vi "Controlling_the_Pump_Reglo_D.vi"(5 "Parameter":string, 7 "Command":T1=enum."Start Reglo Digital", 8 "error in (no error)":errorcluster, 11 "Pumpe":T2=enum."P_01") -> (0 "error out":errorcluster, 3 "Answer":string)   [LabVIEW 2019]
doc: "Contains the commands to controll the Reglo Digital\n\n08.12.2003 - Ismatec/CS"
uses:
  Pumpen.ctl
  Controlling_the_Pump_Reglo_D.ctl
panel:
  in  "VISA resource name In":refnum<visa-resource-name>="COM1"
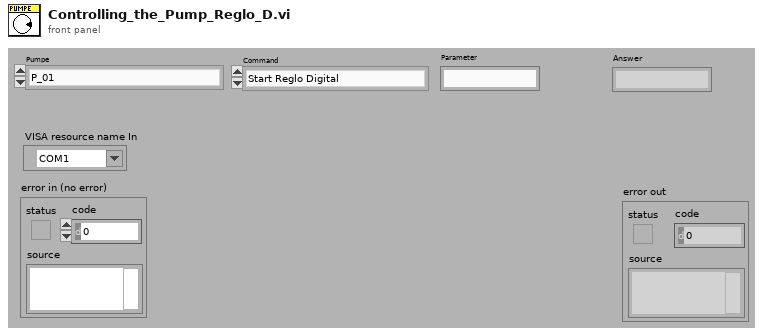
[diagram p1: front panel]
types:
  T1 = typedef "Controlling_the_Pump_Reglo_D.ctl" = enum16{"Reset overload", "Start Reglo Digital", "Stop Reglo Digital", "Revolution Clockwise", "Revolution Counter Clock Wise", "Controlpanel to Manual operation", "Controlpanel Inactiv", "Writing Numbers for Control Panel", "Writing Letters for Controlpanel"}
  T2 = typedef "Pumpen.ctl" = enum16{"Pumpe mit Adresse 0 gibt es nicht", "P_01", "P_02", "P_03", "P_04", "P_05", "P_06", "P_07", "P_08"}
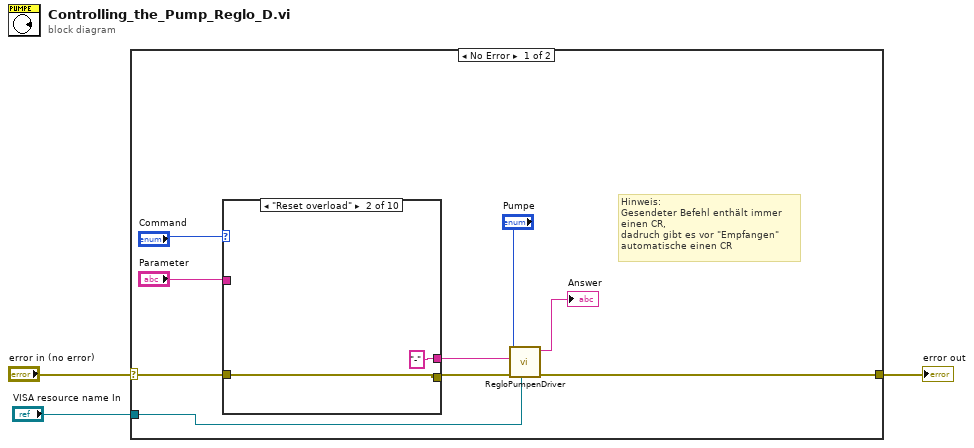
[diagram p0: block diagram]
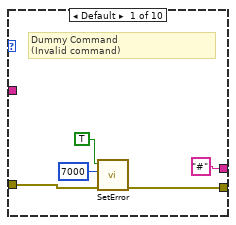
[diagram p2: hidden frame]
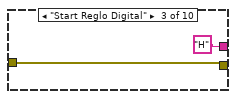
[diagram p3: hidden frame]
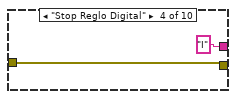
[diagram p4: hidden frame]
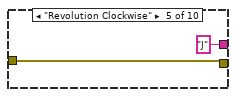
[diagram p5: hidden frame]
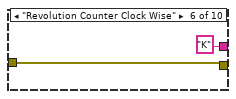
[diagram p6: hidden frame]
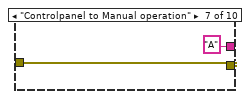
[diagram p7: hidden frame]
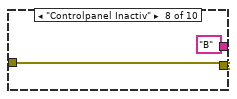
[diagram p8: hidden frame]
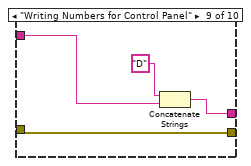
[diagram p9: hidden frame]
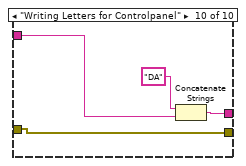
[diagram p10: hidden frame]
diagram:
  n1 = case shown="No Error" "error in (no error)" {
    selector: "error in (no error)" -> [w11 w40]
    tunnel: [w5 w40] -> w2
    tunnel: "VISA resource name In" -> [w4 _]
    frame No Error {
      # "Hinweis:\nGesendeter Befehl enthält immer einen CR,\ndadruch gibt es vor \"Empfangen\"  automatische einen CR"
      n2 = case shown="\"Reset overload\"" "Command" {
        tunnel: [w17 w19 w21 w23 w25 w27 w29 w31 w34 w37] -> w10
        tunnel: w11 -> [w16 w19 w21 w23 w25 w27 w29 w31 w34 w37]
        tunnel: ["#" ("Parameter") "-" ("Parameter") "H" "I" "J" "K" "A" "B" w35 w38] -> w7
        tunnel: "Parameter" -> [_ _ _ _ _ _ _ _ w32 w36]
        frame Default {
          # "Dummy Command\n(Invalid command)"
          n3 = call "SetError.vi"("error in"=w16, "error code"=7000, "Error?"=TRUE) -> ("error out"=w17:errorcluster)  [unwired: 6 in]
        }
        frame "Reset overload" {
        }
        frame "Start Reglo Digital" {
        }
        frame "Stop Reglo Digital" {
        }
        frame "Revolution Clockwise" {
        }
        frame "Revolution Counter Clock Wise" {
        }
        frame "Controlpanel to Manual operation" {
        }
        frame "Controlpanel Inactiv" {
        }
        frame "Writing Numbers for Control Panel" {
          n4 = Concatenate Strings("D" ("String"), w32) -> (w35:string)
        }
        frame "Writing Letters for Controlpanel" {
          n5 = Concatenate Strings("DA" ("String"), w36) -> (w38:string)
        }
      }
      n6 = call "RegloPumpenDriver.vi"("VISA resource name In"=w4, "error in"=w10, "Befehl"=w7, "Pump"="Pumpe") -> ("error out"=w5:errorcluster, "Receivestring"=→"Answer":string)  [unwired: 3 in, 3 out]
    }
    frame Error {
    }
  }
  "error out" <- w2
